vi "CmdData2.vi"() -> ()   [LabVIEW 2011]
panel:
  in  "Data2":dbl
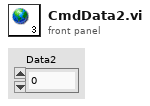
[diagram p1: front panel]
diagram:
